vi "sr400_get_data.vi"(8 "error in (no error)":errorcluster, 10 "Settings In":T2={"Channel A"={"Input"=0, "A Discriminator Level (V)"=0.0, "A Discriminator Slope"=enum."Falling", "A Gate Mode"=enum."CW", "A Gate Delay (s)"=0.0, "A Gate Width (s)"=5e-09, "Scan Increment (s)"=0.0}, "Channel B"={"Input"=0, "B Discriminator Level (V)"=0.0, "B Discriminator Slope"=enum."Falling", "B Gate Mode"=enum."CW", "B Gate Delay (s)"=0.0, "B Gate Width (s)"=5e-09, "Scan Increment (s)"=0.0}, "Channel T"={"Input"=0, "Trigger Level (V)"=0.0, "Trigger Slope"=enum."Falling", "T Discriminator Slope"=enum."Falling", "T Discriminator Level (V)"=0.0, "Trigger Preset"=1.0}, "N Periods"=0.0, "At N"=enum."Stop", "Counting Mode"=enum."A,B for T Preset", "GPIB Address"="", "Dwell Time (s)"=0.002, "Port 1 Mode"=0, "Port 1 Voltage"=0.0, "Port 1 Scan Increment"=-0.5, "Port 2 Voltage"=0.0, "Port 2 Scan Increment"=0.0, "Port 2 Mode"=0, "Counter Toggle"=FALSE, "Pusleblater Settings"={"Loop Start Channel"=0.0, "Loop End Channel"=0.0, "Loop On"=FALSE}} {"Port 2 Mode" items=["Scan"=1, "Fixed"=0]; "Port 2 Scan Increment" min=-0.5 max=0.5; "Port 2 Voltage" min=-10.0 max=10.0; "Port 1 Scan Increment" min=-0.5 max=-0.5; "Port 1 Voltage" min=-10.0 max=10.0; "Port 1 Mode" items=["Scan"=1, "Fixed"=0]; "Dwell Time (s)" min=0.002 max=60.0 format="%#_6p"; "N Periods" min=0.0 max=2000.0 step=1.0; "Channel T"."Trigger Preset" min=1.0 max=900000000000.0 format="%#_1e"; "Channel T"."T Discriminator Level (V)" min=-0.3 max=0.3 format="%#_6p"; "Channel T"."Trigger Level (V)" min=-2.0 max=2.0 format="%#_6p"; "Channel T"."Input" items=["10 MHz", "Input 2", "Trig"]; "Channel B"."Scan Increment (s)" min=0.0 max=0.09992 format="%#_6p"; "Channel B"."B Gate Width (s)" min=5e-09 max=0.9992 format="%#_6p"; "Channel B"."B Gate Delay (s)" min=0.0 max=0.9992 format="%#_6p"; "Channel B"."B Discriminator Level (V)" min=-0.3 max=0.3 format="%#_6p"; "Channel B"."Input" items=["Input 2"=2, "Input 1"=1]; "Channel A"."Scan Increment (s)" min=0.0 max=0.09992 format="%#_6p"; "Channel A"."A Gate Width (s)" min=5e-09 max=0.9992 format="%#_6p"; "Channel A"."A Gate Delay (s)" min=0.0 max=0.9992 format="%#_6p"; "Channel A"."A Discriminator Level (V)" min=-0.3 max=0.3 format="%#_6p"; "Channel A"."Input" items=["Input 1", "10 MHz"]}) -> (0 "error out":errorcluster, 1 "Counter B Data":i32[](array[numeric]), 2 "Counter A Data":i32[](array[numeric]))   [LabVIEW 2013]
uses:
  Controls/SR400/SR400.ctl
  Controls/SR400/Channel A/channelA.ctl
  Controls/SR400/Channel A/channelA_inputs.ctl
  Controls/SR400/discrim_slope.ctl
  Controls/SR400/gate_mode.ctl
  Controls/SR400/Channel B/channelB.ctl
  Controls/SR400/Channel B/inputsB.ctl
  Controls/SR400/Channel T/channelT.ctl
  Controls/SR400/Channel T/inputsT.ctl
  <vilib>/Instr/_visa.llb/GPIB Status Boolean Array.ctl
panel:
  out "ibsta":T1
  out "a string":string[](array[string])
  out "b string":string[](array[string])
  out "Numeric":i32
  out "data 2":string
  out "Settings Out":T2={"Channel A"={"Input"=0, "A Discriminator Level (V)"=0.0, "A Discriminator Slope"=enum."Falling", "A Gate Mode"=enum."CW", "A Gate Delay (s)"=0.0, "A Gate Width (s)"=5e-09, "Scan Increment (s)"=0.0}, "Channel B"={"Input"=0, "B Discriminator Level (V)"=0.0, "B Discriminator Slope"=enum."Falling", "B Gate Mode"=enum."CW", "B Gate Delay (s)"=0.0, "B Gate Width (s)"=5e-09, "Scan Increment (s)"=0.0}, "Channel T"={"Input"=0, "Trigger Level (V)"=0.0, "Trigger Slope"=enum."Falling", "T Discriminator Slope"=enum."Falling", "T Discriminator Level (V)"=0.0, "Trigger Preset"=1.0}, "N Periods"=0.0, "At N"=enum."Stop", "Counting Mode"=enum."A,B for T Preset", "GPIB Address"="", "Dwell Time (s)"=0.002, "Port 1 Mode"=0, "Port 1 Voltage"=0.0, "Port 1 Scan Increment"=-0.5, "Port 2 Voltage"=0.0, "Port 2 Scan Increment"=0.0, "Port 2 Mode"=0, "Counter Toggle"=FALSE, "Pusleblater Settings"={"Loop Start Channel"=0.0, "Loop End Channel"=0.0, "Loop On"=FALSE}} {"Port 2 Mode" items=["Scan"=1, "Fixed"=0]; "Port 2 Scan Increment" min=-0.5 max=0.5; "Port 2 Voltage" min=-10.0 max=10.0; "Port 1 Scan Increment" min=-0.5 max=-0.5; "Port 1 Voltage" min=-10.0 max=10.0; "Port 1 Mode" items=["Scan"=1, "Fixed"=0]; "Dwell Time (s)" min=0.002 max=60.0 format="%#_6p"; "N Periods" min=0.0 max=2000.0 step=1.0; "Channel T"."Trigger Preset" min=1.0 max=900000000000.0 format="%#_1e"; "Channel T"."T Discriminator Level (V)" min=-0.3 max=0.3 format="%#_6p"; "Channel T"."Trigger Level (V)" min=-2.0 max=2.0 format="%#_6p"; "Channel T"."Input" items=["10 MHz", "Input 2", "Trig"]; "Channel B"."Scan Increment (s)" min=0.0 max=0.09992 format="%#_6p"; "Channel B"."B Gate Width (s)" min=5e-09 max=0.9992 format="%#_6p"; "Channel B"."B Gate Delay (s)" min=0.0 max=0.9992 format="%#_6p"; "Channel B"."B Discriminator Level (V)" min=-0.3 max=0.3 format="%#_6p"; "Channel B"."Input" items=["Input 2"=2, "Input 1"=1]; "Channel A"."Scan Increment (s)" min=0.0 max=0.09992 format="%#_6p"; "Channel A"."A Gate Width (s)" min=5e-09 max=0.9992 format="%#_6p"; "Channel A"."A Gate Delay (s)" min=0.0 max=0.9992 format="%#_6p"; "Channel A"."A Discriminator Level (V)" min=-0.3 max=0.3 format="%#_6p"; "Channel A"."Input" items=["Input 1", "10 MHz"]}
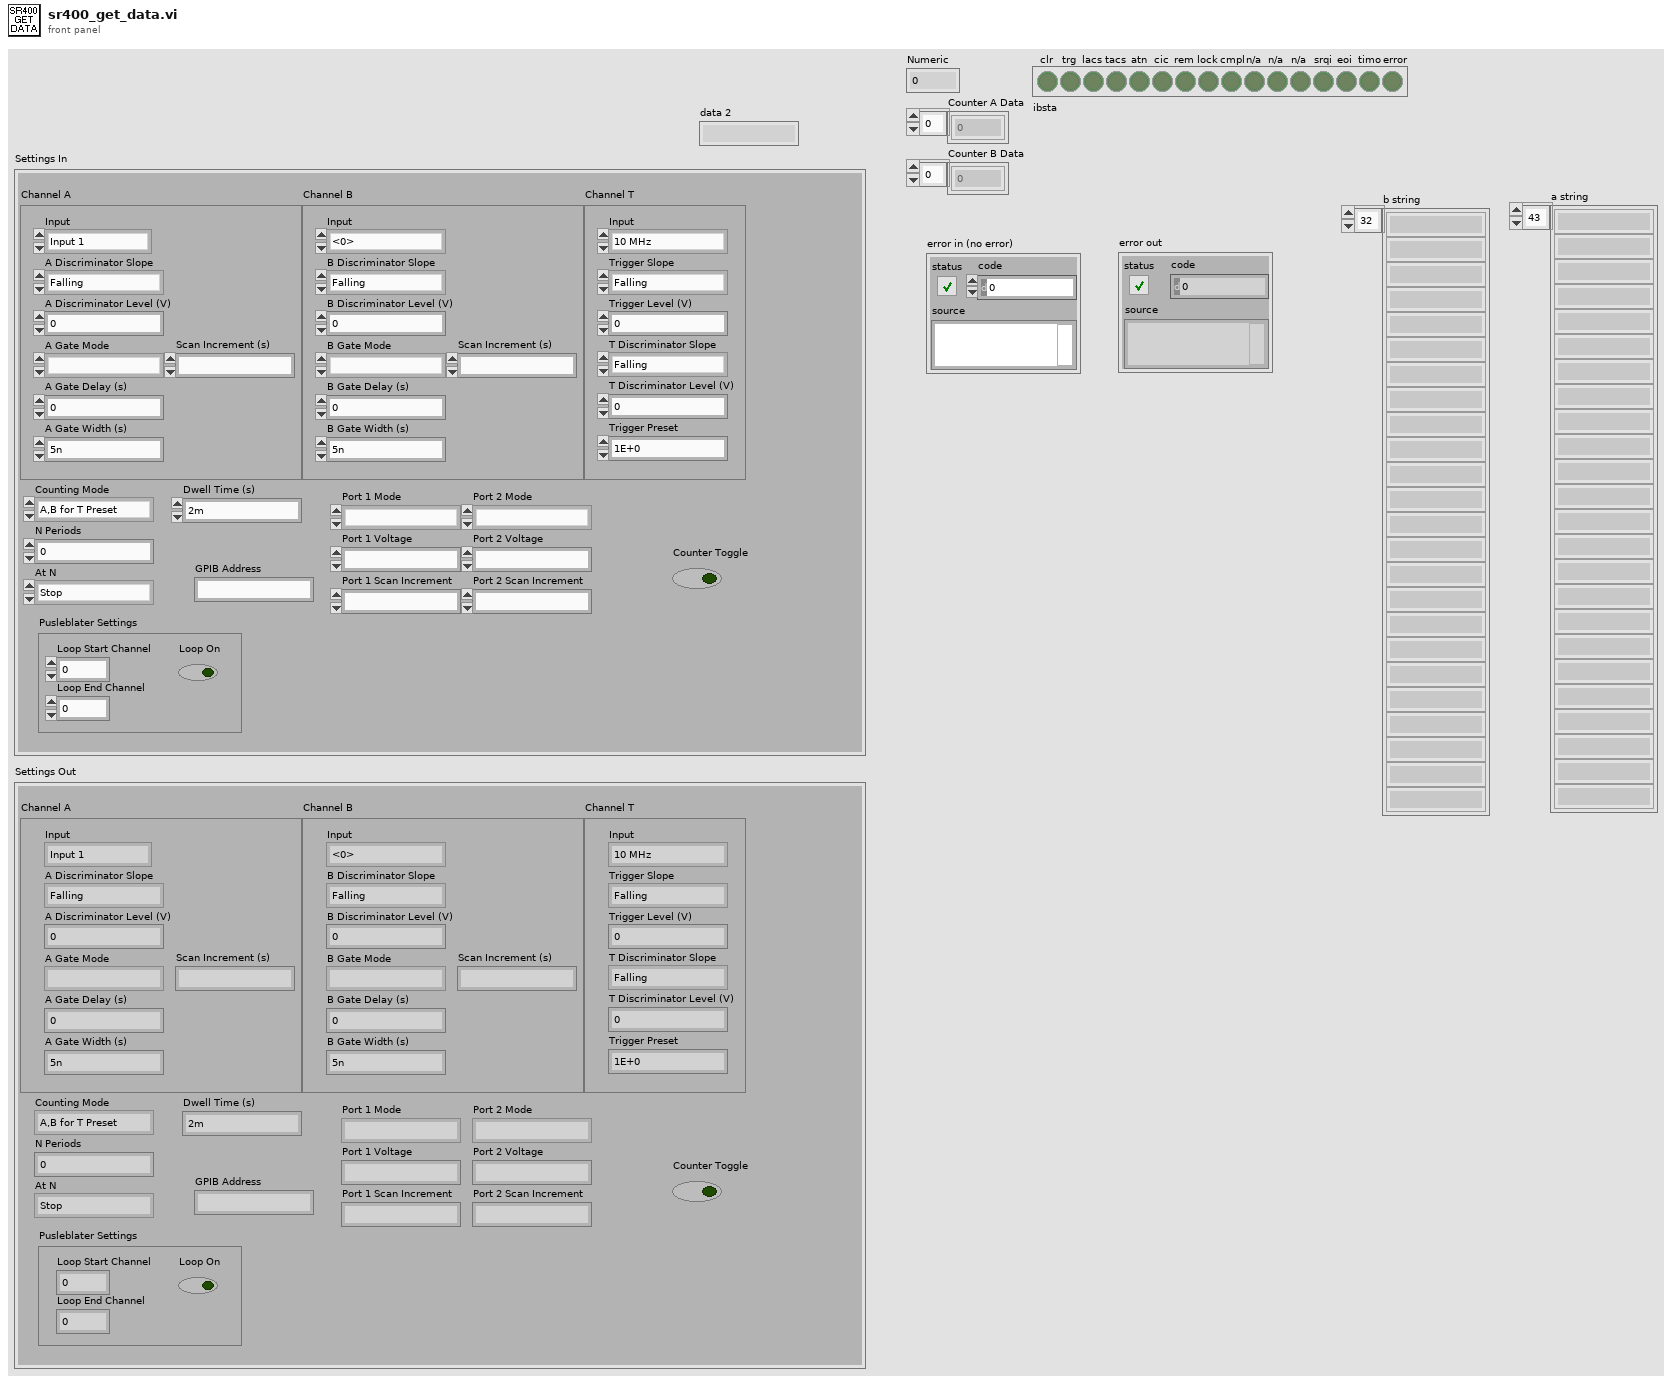
[diagram p1: front panel]
types:
  T1 = typedef "GPIB Status Boolean Array.ctl" = bool[]
  T2 = typedef "SR400.ctl" = cluster{"Channel A":T3, "Channel B":T7, "Channel T":T9, "N Periods":dbl, "At N":enum16{"Stop", "Start"}, "Counting Mode":enum16{"A,B for T Preset", "A-B for T Preset", "A+B for T Preset"}, "GPIB Address":string, "Dwell Time (s)":dbl, "Port 1 Mode":i32, "Port 1 Voltage":dbl, "Port 1 Scan Increment":dbl, "Port 2 Voltage":dbl, "Port 2 Scan Increment":dbl, "Port 2 Mode":i32, "Counter Toggle":bool, "Pusleblater Settings":cluster{"Loop Start Channel":dbl, "Loop End Channel":dbl, "Loop On":bool}}
  T3 = typedef "channelA.ctl" = cluster{"Input":T4, "A Discriminator Level (V)":dbl, "A Discriminator Slope":T5, "A Gate Mode":T6, "A Gate Delay (s)":dbl, "A Gate Width (s)":dbl, "Scan Increment (s)":dbl}
  T4 = typedef "channelA_inputs.ctl" = u16
  T5 = typedef "discrim_slope.ctl" = enum16{"Rising", "Falling"}
  T6 = typedef "gate_mode.ctl" = enum16{"CW", "Fixed", "Scan"}
  T7 = typedef "channelB.ctl" = cluster{"Input":T8, "B Discriminator Level (V)":dbl, "B Discriminator Slope":T5, "B Gate Mode":T6, "B Gate Delay (s)":dbl, "B Gate Width (s)":dbl, "Scan Increment (s)":dbl}
  T8 = typedef "inputsB.ctl" = u16
  T9 = typedef "channelT.ctl" = cluster{"Input":T10, "Trigger Level (V)":dbl, "Trigger Slope":T5, "T Discriminator Slope":T5, "T Discriminator Level (V)":dbl, "Trigger Preset":dbl}
  T10 = typedef "inputsT.ctl" = u16
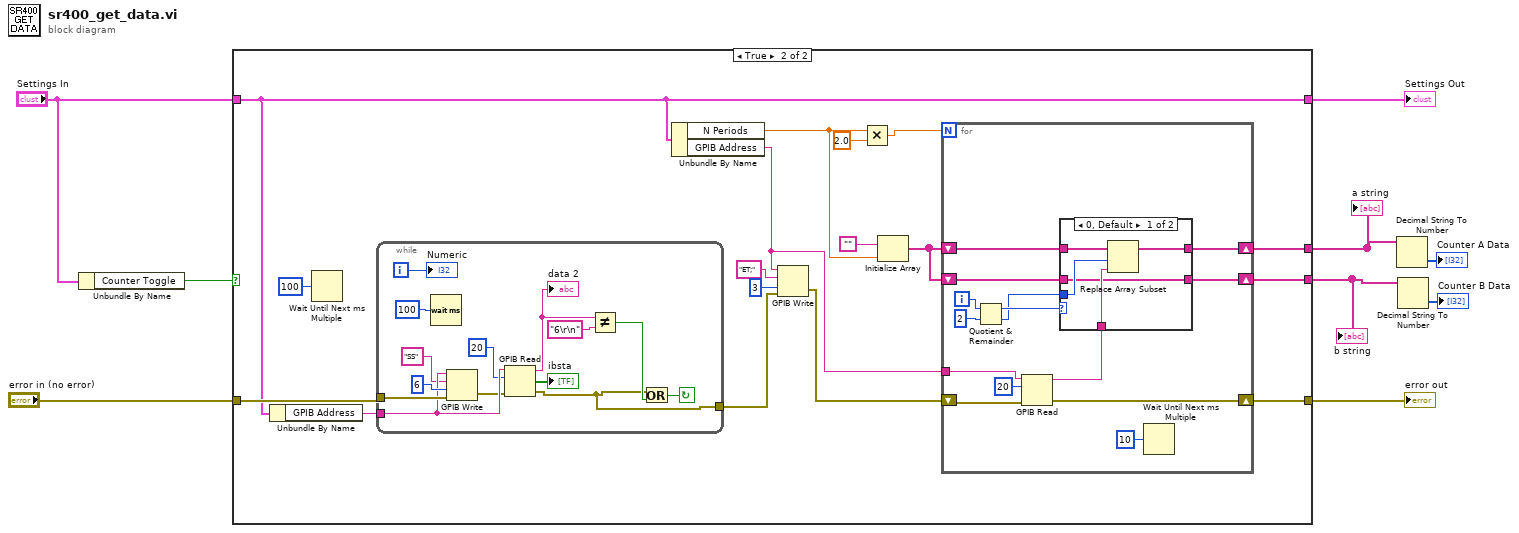
[diagram p0: block diagram]
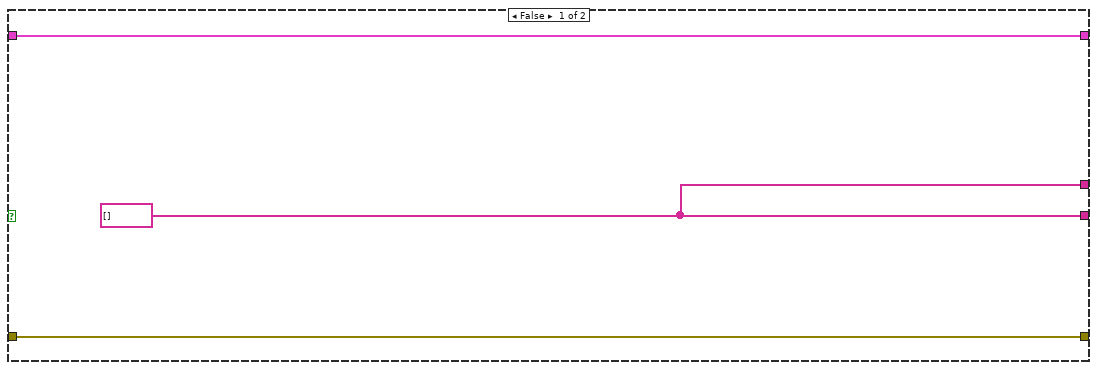
[diagram p2: hidden frame]
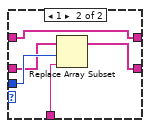
[diagram p3: hidden frame]
diagram:
  n1 = Unbundle By Name("Settings In") -> ("Counter Toggle"=w5:bool)
  n2 = case shown="True" w5 {
    tunnel: "error in (no error)" -> [w10 w27]
    tunnel: "Settings In" -> [w11 w18]
    tunnel: [w10 w23] -> w7
    tunnel: [w9 w20] -> w4
    tunnel: [w9 w19] -> w3
    tunnel: [w11 w18] -> _
    frame False {
      w9 = string[] []
    }
    frame True {
      n3 = Unbundle By Name(w18) -> ("GPIB Address"=w28:string)
      n4 = Wait Until Next ms Multiple(millisecond multiple=u32 100) -> ()  [unwired: 1 out]
      n5 = while {
        tunnel: w28 -> [w63]
        tunnel: w27 -> [w64]
        tunnel: [w53] -> w15
        i -> [w58]
        stop <- w65 continue-if-true
        n6 = Wait (ms)(milliseconds to wait=u32 100 ("millisecond multiple")) -> ()  [unwired: 1 out]
        n7 = GPIB Write(0:w63, 1:"SS", 2:i16 6 ("mode (0)"), 3:w64) -> (6:w61:errorcluster)  [unwired: 1 in, 1 out]
        n8 = GPIB Read(0:w63, 1:20 ("byte count"), 3:w61) -> (5:w56:string, 6:→"ibsta":bool[], 7:w53:errorcluster)  [unwired: 2 in]
        "data 2" <- w56
        n9 = Not Equal?(x=w56, y="6\r\n") -> (x != y?=w54:bool)
        n10 = Or(x=w53, y=w54) -> (x .or. y?=w65:bool)
        "Numeric" <- w58
      }
      n11 = Unbundle By Name(w18) -> ("N Periods"=w14:dbl, "GPIB Address"=w17:string)
      n12 = GPIB Write(0:w17, 1:"ET;" ("data"), 2:i16 3 ("mode (0)"), 3:w15) -> (6:w16:errorcluster)  [unwired: 1 in, 1 out]
      n13 = Multiply(x=w14, y=2.0) -> (x*y=w13:dbl)
      n14 = Initialize Array("", w14) -> (w21:string[])
      n15 = for {
        N: w13 -> [_]
        tunnel: w17 -> [w42]
        shift-right: [w34] -> w20
        shift-left: w21 -> [w33]
        shift-right: [w31] -> w19
        shift-left: w21 -> [w30]
        shift-right: [w37] -> w23
        shift-left: w16 -> [w38]
        i -> [w40]
        n16 = Quotient & Remainder(x=w40, y=2) -> (x-y*floor(x/y)=w36:i32, floor(x/y)=w35:i32)
        n17 = GPIB Read(0:w42, 1:20 ("byte count"), 3:w38) -> (5:w32:string, 7:w37:errorcluster)  [unwired: 2 in, 1 out]
        n18 = case shown="0, Default" w36 {
          tunnel: w35 -> [w44 w51]
          tunnel: [w45 w48] -> w34
          tunnel: w33 -> [w46 w48]
          tunnel: w32 -> [w47 w52]
          tunnel: [w43 w49] -> w31
          tunnel: w30 -> [w43 w50]
          frame 0, Default {
            n19 = Replace Array Subset(array=w46, new element=w47, index=w44) -> (w45:string[])
          }
          frame 1 {
            n20 = Replace Array Subset(array=w50, new element=w52, index=w51) -> (w49:string[])
          }
        }
        n21 = Wait Until Next ms Multiple(millisecond multiple=u32 10) -> ()  [unwired: 1 out]
      }
    }
  }
  "error out" <- w7
  "b string" <- w3
  "a string" <- w4
  n22 = Decimal String To Number(string=w4) -> (number=→"Counter A Data":i32[])  [unwired: 2 in, 1 out]
  n23 = Decimal String To Number(string=w3) -> (number=→"Counter B Data":i32[])  [unwired: 2 in, 1 out]
  "Settings Out" <- "Settings In"
